vi "run.vi"(8 "error in (no error)":errorcluster, 11 "HGF_Monitor in":refnum<class "HGF_Monitor.lvclass">) -> (0 "error out":errorcluster, 3 "HGF_Monitor out":refnum<class "HGF_Monitor.lvclass">)   [LabVIEW 2012, in "HGF_SV.lvlib" / "HGF_Monitor.lvclass"]
uses:
  HGF_Monitor.lvclass
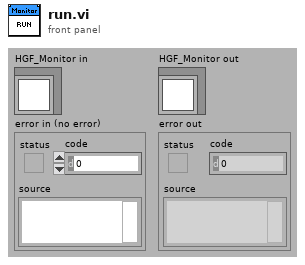
[diagram p1: front panel]
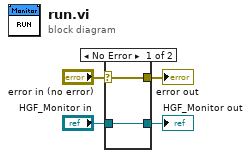
[diagram p0: block diagram]
diagram:
  n1 = case shown="No Error" "error in (no error)" {
    selector: "error in (no error)" -> [w5 w8]
    tunnel: [w5 w8] -> w3
    tunnel: [w6 w7] -> w1
    tunnel: "HGF_Monitor in" -> [w6 w7]
    frame No Error {
    }
    frame Error {
    }
  }
  "error out" <- w3
  "HGF_Monitor out" <- w1
